vi "Core-InitializeQueues.vi"(6 "Cmd(Initialize)":enum16{"Initialize", "UnInitialize"}(ring), 8 "ErrI(No Error)":errorcluster) -> (0 "ErrO":errorcluster, 1 "ErrQRef":refnum<queue>, 2 "DaqQRef":refnum<queue>, 3 "MainQRef":refnum<queue>)   [LabVIEW 2021]
doc: "Initialize or Uninitialize the Queues.\n- if \"Cmd\" was set to \"Initialize\", the Main/DAQ/Error Queues will be created and initialized;\n- if \"Cmd\" was set to \"UnInitialize\", the vi will delete all elements and then destroy the Main/DAQ/Error Queues;\n\nNotes:\n- You can add code here if you want to add more loop in framework."
panel:
  # "Inputs"
  # "Outputs"
  # ":: Modularized Parallism Templete ::\n- Main State Machine -\nby: Gaoke Yang <gaoke.yang@yahoo.com>\nhttp://www.mViAcademy.com\nCopyright (C) 2010, mVi Academy All Rights Reserved"
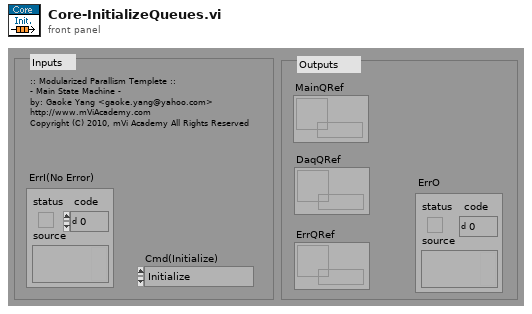
[diagram p1: front panel]
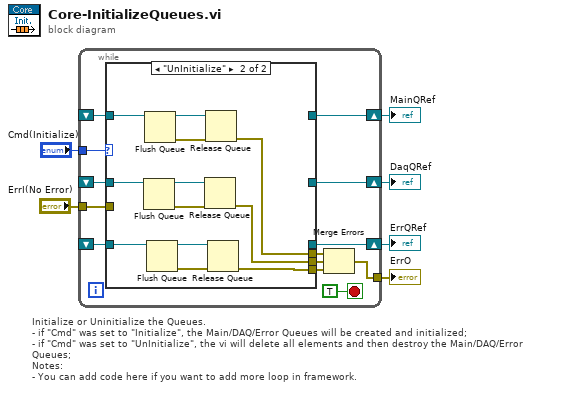
[diagram p0: block diagram]
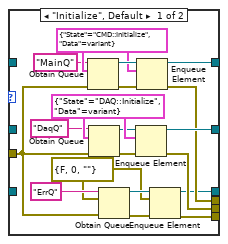
[diagram p2: hidden frame]
diagram:
  # "Initialize or Uninitialize the Queues.\n- if \"Cmd\" was set to \"Initialize\", the Main/DAQ/Error Queues will be created and initialized;\n- if \"Cmd\" was set to \"UnInitialize\", the vi will delete all elements and then destroy the Main/DAQ/Error Queues;\nNotes:\n- You can add code here if you want to add more loop in framework."
  n1 = while {
    tunnel: [w10] -> w4
    tunnel: "ErrI(No Error)" -> [w17]
    shift-right: [w18] -> w5
    shift-left: _ -> [w14]
    shift-right: [w19] -> w6
    shift-left: _ -> [w13]
    tunnel: "Cmd(Initialize)" -> [w15]
    shift-right: [w9] -> w1
    shift-left: _ -> [w7]
    stop <- TRUE stop-if-true
    n2 = case shown="\"UnInitialize\"" w15 {
      tunnel: [w30 _] -> w19
      tunnel: [w29 _] -> w18
      tunnel: w17 -> [w23 _]
      tunnel: w14 -> [_ w50]
      tunnel: w13 -> [_ w45]
      tunnel: [w28 w44] -> w12
      tunnel: [w27 w43] -> w11
      tunnel: [w21 _] -> w9
      tunnel: [w20 w39] -> w8
      tunnel: w7 -> [_ w41]
      frame "Initialize", Default {
        w22 = errorcluster {"status"=FALSE, "code"=0, "source"=""} ("error in (no error)")
        w35 = cluster{"State":string, "Data":variant} {"State"="DAQ::Initialize", "Data"=variant} ("DaqQueue")
        w36 = cluster{"State":string, "Data":variant} {"State"="CMD::Initialize", "Data"=variant} ("MainQueue")
        n3 = Obtain Queue(name (unnamed)="MainQ", element data type=w36, error in (no error)=w23) -> (queue out=w38:refnum<queue>, error out=w37:errorcluster)  [unwired: 2 in, 1 out]
        n4 = Obtain Queue(name (unnamed)="DaqQ", element data type=w35, error in (no error)=w23) -> (queue out=w33:refnum<queue>, error out=w34:errorcluster)  [unwired: 2 in, 1 out]
        n5 = Obtain Queue(name (unnamed)="ErrQ", element data type=w22, error in (no error)=w23) -> (queue out=w25:refnum<queue>, error out=w24:errorcluster)  [unwired: 2 in, 1 out]
        n6 = Enqueue Element(queue=w33, element=w35, error in (no error)=w34) -> (queue out=w30:refnum<queue>, error out=w27:errorcluster)  [unwired: 2 out]
        n7 = Enqueue Element(queue=w38, element=w36, error in (no error)=w37) -> (queue out=w29:refnum<queue>, error out=w28:errorcluster)  [unwired: 2 out]
        n8 = Enqueue Element(queue=w25, element=w22, error in (no error)=w24) -> (queue out=w21:refnum<queue>, error out=w20:errorcluster)  [unwired: 2 out]
      }
      frame "UnInitialize" {
        n9 = Flush Queue(queue=w45) -> (queue out=w46:refnum<queue>, error out=w47:errorcluster)  [unwired: 1 in, 1 out]
        n10 = Flush Queue(queue=w50) -> (queue out=w49:refnum<queue>, error out=w48:errorcluster)  [unwired: 1 in, 1 out]
        n11 = Flush Queue(queue=w41) -> (queue out=w42:refnum<queue>, error out=w40:errorcluster)  [unwired: 1 in, 1 out]
        n12 = Release Queue(queue=w46, error in (no error)=w47) -> (error out=w43:errorcluster)  [unwired: 1 in, 2 out]
        n13 = Release Queue(queue=w49, error in (no error)=w48) -> (error out=w44:errorcluster)  [unwired: 1 in, 2 out]
        n14 = Release Queue(queue=w42, error in (no error)=w40) -> (error out=w39:errorcluster)  [unwired: 1 in, 2 out]
      }
    }
    n15 = Merge Errors(w12, w11, w8) -> (w10:errorcluster)
  }
  "ErrO" <- w4
  "MainQRef" <- w5
  "DaqQRef" <- w6
  "ErrQRef" <- w1
